vi "CreateRotationZ.vi"(8 "error in (no error)":errorcluster, 9 "radians":dbl, 11 "3D Scene in":refnum<class "3D Scene.lvclass">) -> (0 "error out":errorcluster, 2 "Modelview out":dbl[][](array[numeric]), 3 "3D Scene out":refnum<class "3D Scene.lvclass">)   [LabVIEW 2015, in "3D Scene.lvclass"]
uses:
  3D Scene.lvclass
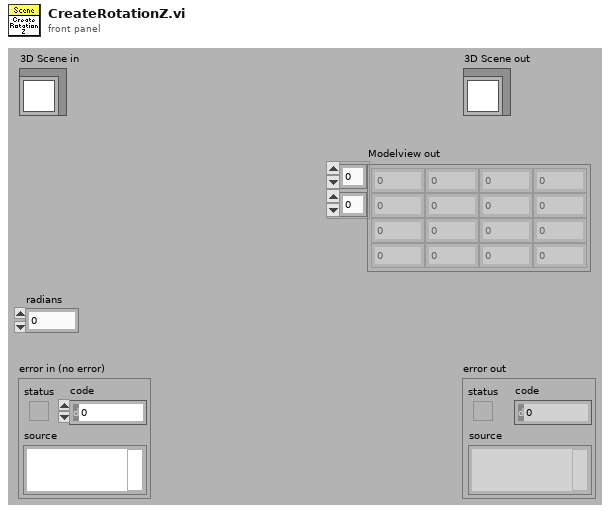
[diagram p1: front panel]
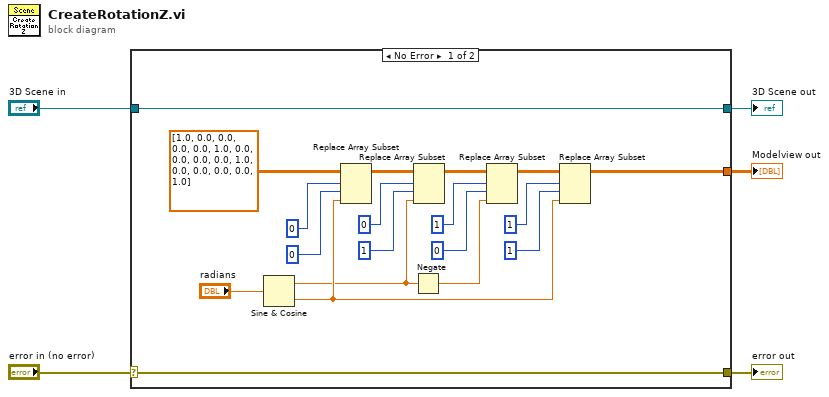
[diagram p0: block diagram]
diagram:
  n1 = case shown="No Error" "error in (no error)" {
    selector: "error in (no error)" -> [w23 w26]
    tunnel: [w23 w26] -> w4
    tunnel: [w24 w25] -> w2
    tunnel: "3D Scene in" -> [w24 w25]
    tunnel: [w7 _] -> w1
    frame No Error {
      n2 = Sine & Cosine(0:"radians") -> (1:w19:dbl, 2:w21:dbl)
      n3 = Replace Array Subset(array=dbl[][] [[1.0, 0.0, 0.0, 0.0], [0.0, 1.0, 0.0, 0.0], [0.0, 0.0, 1.0, 0.0], [0.0, 0.0, 0.0, 1.0]], new element=w21, index (row)=0, index (col)=0 ("disabled index (col)")) -> (w8:dbl[][])
      n4 = Negate(x=w19) -> (-x=w20:dbl)
      n5 = Replace Array Subset(array=w8, new element=w19, index (row)=0 ("disabled index (row)"), index (col)=1 ("disabled index (col)")) -> (w9:dbl[][])
      n6 = Replace Array Subset(array=w9, new element=w20, index (row)=1, index (col)=0 ("disabled index (col)")) -> (w10:dbl[][])
      n7 = Replace Array Subset(array=w10, new element=w21, index (row)=1, index (col)=1 ("disabled index (col)")) -> (w7:dbl[][])
    }
    frame Error {
    }
  }
  "error out" <- w4
  "3D Scene out" <- w2
  "Modelview out" <- w1
